vi "Find Widest Gap.vi"(11 "Blocked Columns":bool[](array[boolean])) -> (3 "Best Known Gap (mm)":cluster{i32, i32})   [LabVIEW 2017]
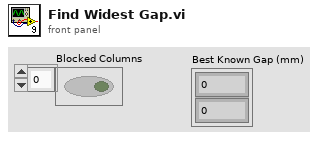
[diagram p1: front panel]
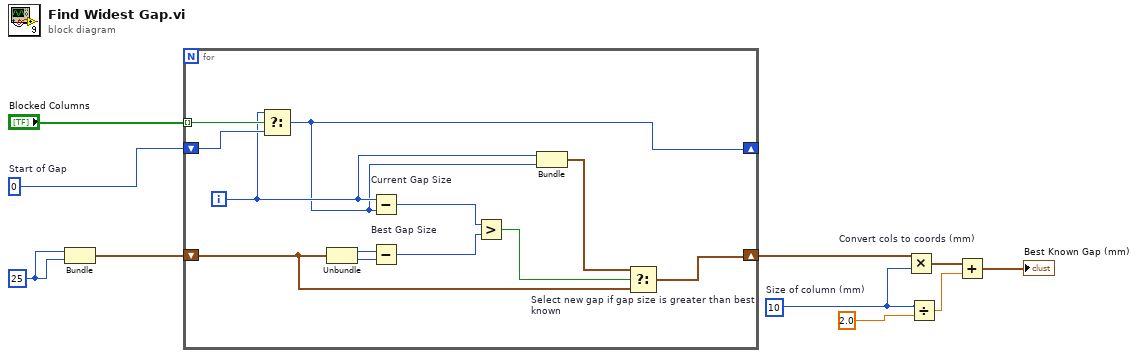
[diagram p0: block diagram]
diagram:
  w5 = 10  # Size of column (mm)
  w7 = 0  # Start of Gap
  w10 = 25
  n1 = Bundle(w10, w10) -> (w8:cluster{i32, i32})  [unwired: 1 in]
  n2 = for {
    tunnel: "Blocked Columns" -> [w15] mode=indexing
    shift-right: [w18] -> w6
    shift-left: w8 -> [w19]
    shift-right: [w11] -> _
    shift-left: w7 -> [w14]
    i -> [w12]
    n3 = Select(t=w12, s=w15, f=w14) -> (s? t:f=w11:i32)
    n4 = Unbundle(w19) -> (w21:i32, w22:i32)
    n5 = Subtract "Current Gap Size"(x=w12, y=w11) -> (x-y=w17:i32)
    n6 = Subtract "Best Gap Size"(x=w21, y=w22) -> (x-y=w16:i32)
    n7 = Greater?(x=w17, y=w16) -> (0:w13:bool)
    n8 = Bundle(w12, "Start of Gap"=w11) -> (w20:cluster{i32, "Start of Gap":i32})  [unwired: 1 in]
    n9 = Select "Select new gap if gap size is greater than best known"(t=w20, s=w13, f=w19) -> (s? t:f=w18:cluster{i32, "Start of Gap":i32})
  }
  n10 = Multiply "Convert cols to coords (mm)"(x=w6, y=w5) -> (x*y=w2:cluster{i32, i32})
  n11 = Divide(x=w5, y=2.0) -> (x/y=w3:dbl)
  n12 = Add(x=w2, y=w3) -> (x+y=→"Best Known Gap (mm)":cluster{dbl, dbl})
